vi "Monitor.vi"(8 "error in (no error)":errorcluster, 10 "PCL Rate (secs)":dbl, 11 "Frame Configurations":T1[](array[typedef]) {"Validation Channels Refs"."Data Reference" format="%.0x"; "CD Results Refs"."Data Reference" format="%.0x"; "Input Channels Refs"."Data Reference" format="%.0x"; "Frame Configuration"."CRC"."Data Type" items=["Signed", "Unsigned", "IEEE Float"]; "Frame Configuration"."Rolling Counter"."Data Type" items=["Signed", "Unsigned", "IEEE Float"]; "Frame Configuration"."Input Channels"."Data Type" items=["Signed", "Unsigned", "IEEE Float"]}) -> (0 "error out":errorcluster, 3 "Frame Configurations":T1[](array[typedef]) {"Validation Channels Refs"."Data Reference" format="%.0x"; "CD Results Refs"."Data Reference" format="%.0x"; "Input Channels Refs"."Data Reference" format="%.0x"; "Frame Configuration"."CRC"."Data Type" items=["Signed", "Unsigned", "IEEE Float"]; "Frame Configuration"."Rolling Counter"."Data Type" items=["Signed", "Unsigned", "IEEE Float"]; "Frame Configuration"."Input Channels"."Data Type" items=["Signed", "Unsigned", "IEEE Float"]})   [LabVIEW 2015, in "Protection and Rolling Counter Addon Engine.lvlib"]
uses:
  Protection and Rolling Counter Addon Engine.lvlib
  Types/RT Engine Monitor References.ctl
  Shared/Types/FrameConfiguration.ctl
  Shared/Types/InputChannelConfiguration.ctl
  Shared/Types/Protection Type.ctl
  <vilib>/NI Veristand/Custom Device API/Block Data Reference.ctl
  <vilib>/NI Veristand/Custom Device API/Data Reference.ctl
  <vilib>/NI Veristand/Custom Device API/Global Data Refs.vi
  <vilib>/NI Veristand/Custom Device API/Custom Device API.lvlib
  Shared/Protection and Rolling Counter Addon Shared.lvlib
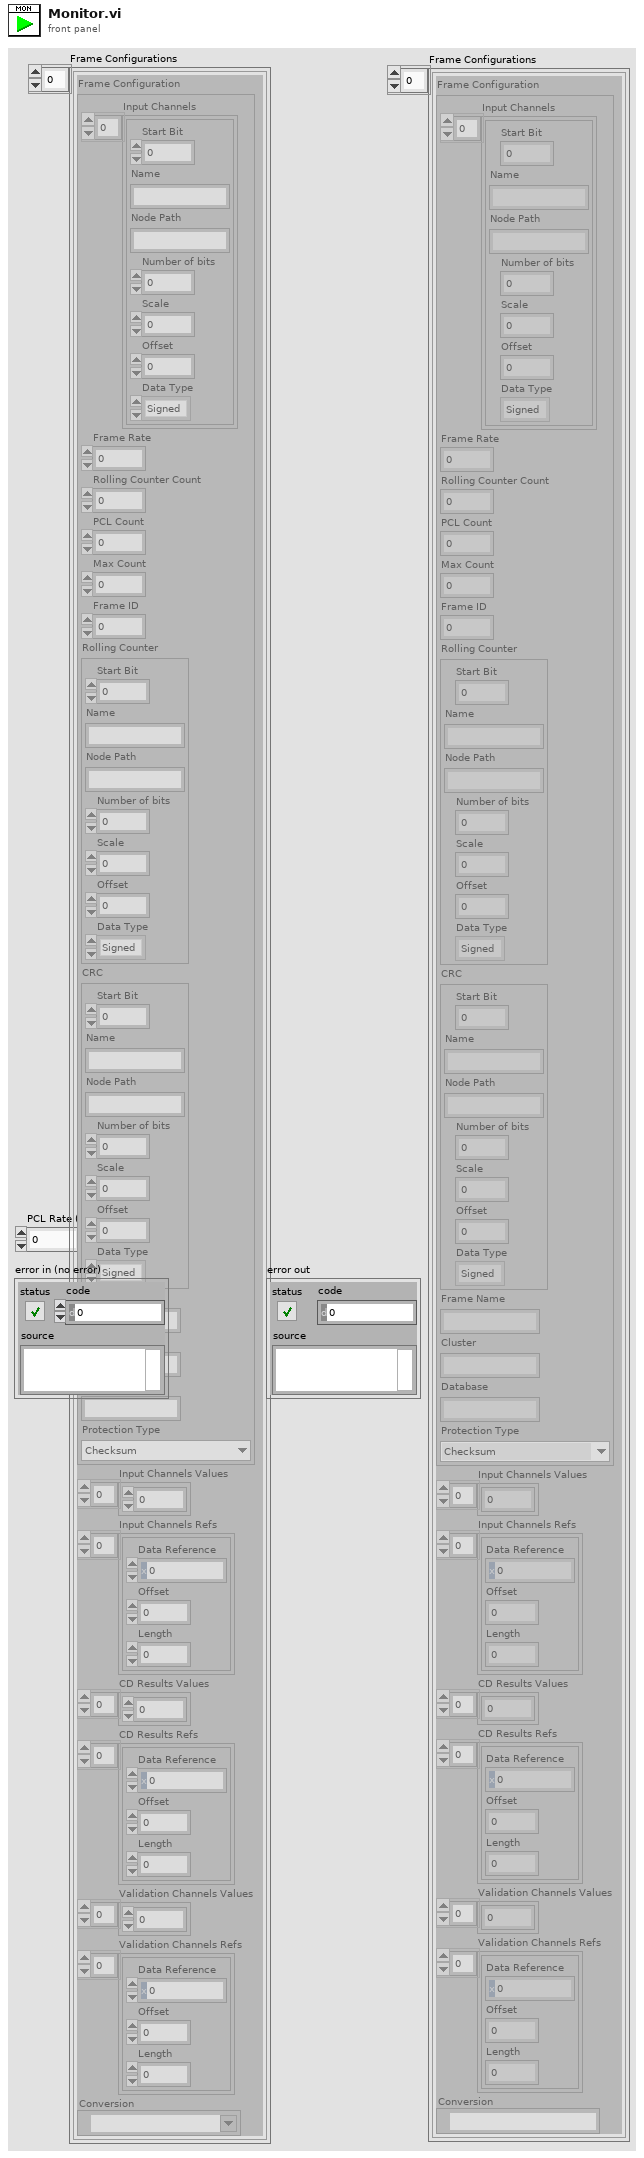
[diagram p1: front panel]
types:
  T1 = typedef "Protection and Rolling Counter Addon Engine.lvlib/RT Engine Monitor References.ctl" = cluster{"Frame Configuration":T2, "Input Channels Values":dbl[], "Input Channels Refs":T5[], "CD Results Values":dbl[], "CD Results Refs":T5[], "Validation Channels Values":dbl[], "Validation Channels Refs":T5[], "Conversion":refnum<k21>}
  T2 = typedef "Protection and Rolling Counter Addon Shared.lvlib/FrameConfiguration.ctl" = cluster{"Input Channels":T3[], "Frame Rate":dbl, "Rolling Counter Count":dbl, "PCL Count":u64, "Max Count":dbl, "Frame ID":u32, "Rolling Counter":T3, "CRC":T3, "Frame Name":string, "Cluster":string, "Database":string, "Protection Type":T4}
  T3 = typedef "Protection and Rolling Counter Addon Shared.lvlib/InputChannelConfiguration.ctl" = cluster{"Start Bit":i32, "Name":string, "Node Path":string, "Number of bits":i32, "Scale":dbl, "Offset":dbl, "Data Type":u32}
  T4 = typedef "Protection and Rolling Counter Addon Shared.lvlib/Protection Type.ctl" = enum16{"Checksum", "CRC", "None (Counter Only)"}
  T5 = typedef "Custom Device API.lvlib/Block Data Reference.ctl" = cluster{"Data Reference":T6, "Offset":u64, "Length":u64}
  T6 = typedef "Custom Device API.lvlib/Data Reference.ctl" = i32
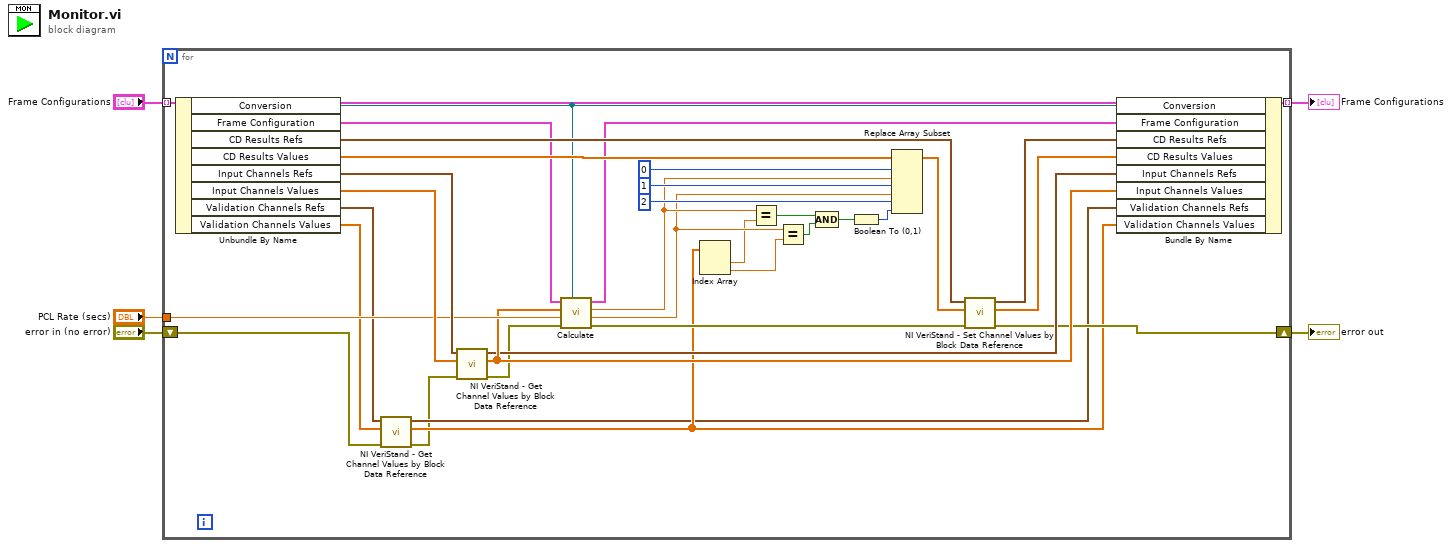
[diagram p0: block diagram]
diagram:
  n1 = for {
    tunnel: "Frame Configurations" -> [w37] mode=indexing
    tunnel: "PCL Rate (secs)" -> [w38]
    shift-right: [w27] -> w2
    shift-left: "error in (no error)" -> [w8]
    tunnel: [w26] -> w4 mode=indexing
    n2 = Unbundle By Name(w37) -> ("Conversion"=w6:refnum<k21>, "Frame Configuration"=w15:T2, "CD Results Refs"=w35:T5[], "CD Results Values"=w36:dbl[], "Input Channels Refs"=w39:T5[], "Input Channels Values"=w40:dbl[], "Validation Channels Refs"=w13:T5[], "Validation Channels Values"=w12:dbl[])
    n3 = call <vilib>:"NI VeriStand - Get Channel Values by Block Data Reference.vi"("error in (no error)"=w8, "Values Array in"=w12, "Block Data Ref"=w13) -> ("error out"=w7:errorcluster, "Values Array out"=w11:dbl[], "Block Data Ref dup"=w10:T5[])  [unwired: 6 in]
    n4 = call <vilib>:"NI VeriStand - Get Channel Values by Block Data Reference.vi"("error in (no error)"=w7, "Values Array in"=w40, "Block Data Ref"=w39) -> ("error out"=w9:errorcluster, "Values Array out"=w29:dbl[], "Block Data Ref dup"=w28:T5[])  [unwired: 6 in]
    n5 = call "Calculate.vi"("Conversion"=w6, "error in (no error)"=w9, "PCL dt"=w38, "Values"=w29, "Frame Configuration"=w15) -> ("error out"=w25:errorcluster, "ProtectionValue"=w18:dbl, "Rolling Counter"=w19:dbl, "Frame Configuration"=w14:T2)  [unwired: 3 in]
    n6 = Index Array(array=w11) -> (element #1=w17:dbl, element #2=w16:dbl)  [unwired: 2 in]
    n7 = Equal?(x=w19, y=w17) -> (x = y?=w23:bool)
    n8 = Equal?(x=w18, y=w16) -> (x = y?=w22:bool)
    n9 = Compound Arithmetic op=AND(w23, w22) -> (w21:bool)
    n10 = Boolean To (0,1)(Boolean=w21) -> (0, 1=w20:i16)
    n11 = Replace Array Subset(array=w36, new element #1=w19, index #1=0 ("index"), new element #2=w18, index #2=1 ("index"), new element #3=w20, index #3=2 ("index")) -> (w34:dbl[])
    n12 = call <vilib>:"NI VeriStand - Set Channel Values by Block Data Reference.vi"("error in (no error)"=w25, "Values Array in"=w34, "Block Data Ref"=w35) -> ("error out"=w27:errorcluster, "Values Array out"=w30:dbl[], "Block Data Ref dup"=w31:T5[])  [unwired: 6 in]
    n13 = Bundle By Name(cluster=w37, "Conversion"=w6, "Frame Configuration"=w14, "CD Results Refs"=w31, "CD Results Values"=w30, "Input Channels Refs"=w28, "Input Channels Values"=w29, "Validation Channels Refs"=w10, "Validation Channels Values"=w11) -> (w26:T1)
  }
  "Frame Configurations" <- w4
  "error out" <- w2
